vi "PrefDialog.vi"(8 "error in (no error)":errorcluster, 11 "MyPluginsBase in":refnum<class "PacificPowerSource.lvclass">) -> (0 "error out":errorcluster, 1 "Save As":bool, 2 "Changed":bool, 3 "MyPluginsBase out":refnum<class "PacificPowerSource.lvclass">)   [LabVIEW 2018, in "AcPwrPlugins.lvlib" / "PacificPowerSource.lvclass"]
doc: "This VI allows the user to display the previous instrument's settings, change these settings, and save the current settings to the same file or a new file with a new \"Type\" identifier."
uses:
  PacificPowerSource.lvclass
  C:/Program Files (x86)/National Instruments/LabVIEW 2018/user.lib/NIST/BaseClasses/BasePlugin_class/BasePlugin.lvclass
  C:/Users/ico/Documents/Projects/NistPluggableModules/AcPwr/AcPwrPlugins/AcPwrBaseClass/AcPwrBase.lvclass
  TypeDefs/Device(s)Settings.ctl
  AcPwrBaseClass/TypeDefs/BaseMeasurements.ctl
  ChromaAcLoadClass/TypeDefs/MeasurementType.ctl
  TypeDefs/Measurements.ctl
  TypeDefs/MeasurementType.ctl
  <userlib>/NIST/BaseClasses/BasePlugin_class/BasePlugin.lvclass/BasePlugin.ctl
  AcPwrBaseClass/AcPwrBase.lvclass/AcPwrBase.ctl
  <userlib>/NIST/BaseClasses/BasePlugin_class/Accessors/Read PluginIniFilePath.vi
  AcPwrBaseClass/Accessors/Read BaseConfig.vi
  AcPwrBaseClass/Accessors/Read BaseMeasurements.vi
  <userlib>/NIST/BaseClasses/BasePlugin_class/Accessors/Write PluginIniFilePath.vi
  <vilib>/Utility/config.llb/NI_LVConfig.lvlib
  AcPwrBaseClass/AcPwrBase.lvclass
  ChromaAcLoadClass/ChromaAcLoad.lvclass
panel:
  in  "Measurements":T1
  in  "BaseMeasurements":T3 {"NHRGridSim Phase" items=["All", "A Phase", "B Phase", "C Phase"]; "NHRDC Measurement Type" items=["Voltage"=1, "Positive Peak Voltage"=2, "Positive Peak Voltage Last Fetch"=4, "Negative Peak Voltage"=8, "Negative Peak Voltage Last Fetch"=16, "Current"=32, "Positive Peak Current"=64, "Positive Peak Current Last Fetch"=128, "Negative Peak Current"=256, "Negative Peak Current Last Fetch"=512, "Power"=1024, "Positive Peak Power"=2048, "Positive Peak Power Last Fetch"=4096, "Negative Peak Power"=8192, "Negative Peak Power Last Fetch"=16384, "Timestamp"=32768, "Charge Time"=65536, "Discharge Time"=131072, "Amp Hour"=262144, "Amp Hour Time"=524288, "Amp Hour Charge"=1048576, "Amp Hour Discharge"=2097152, "Kilo Watt Hour"=4194304, "Kilo Watt Hour Time"=8388608, "Kilo Watt Hour Charge"=16777216, "Kilo Watt Hour Discharge"=33554432, "UUT Temperature"=67108864]; "NHRDC Fetch Method" items=["Aperture", "Immediate"]}
  in  "btnSaveAs":bool
  in  "Measurement RefreshTime (ms)":u32
  in  "btnSave":bool
  in  "btnCancel":bool
  in  "Device(s)Settings":T5 {"Modules"."Source Range"."Frequency Range (600Hz)" items=["150 Hz", "300 Hz", "600 Hz", "1200 Hz"]; "Modules"."Source Range"."Range Control (0: Auto)" items=["Auto", "<110 V", "110 V -120.9 V", "121 V - 130.9 V", "> 131 V"]; "Modules"."Program #"."Waveform C (1: Sine)" items=["Sine"=1, "Arbitrary Waveform 2"=2, "Arbitrary Waveform 3"=3, "Arbitrary Waveform 4"=4, "Arbitrary Waveform 5"=5, "Arbitrary Waveform 6"=6, "Arbitrary Waveform 7"=7, "Arbitrary Waveform 8"=8, "Arbitrary Waveform 9"=9, "Arbitrary Waveform 10"=10, "Arbitrary Waveform 11"=11, "Arbitrary Waveform 12"=12, "Arbitrary Waveform 13"=13, "Arbitrary Waveform 14"=14, "Arbitrary Waveform 15"=15, "Arbitrary Waveform 16"=16, "Arbitrary Waveform 17"=17, "Arbitrary Waveform 18"=18, "Arbitrary Waveform 19"=19, "Arbitrary Waveform 20"=20, "Arbitrary Waveform 21"=21, "Arbitrary Waveform 22"=22]; "Modules"."Program #"."Waveform B (1: Sine)" items=["Sine"=1, "Arbitrary Waveform 2"=2, "Arbitrary Waveform 3"=3, "Arbitrary Waveform 4"=4, "Arbitrary Waveform 5"=5, "Arbitrary Waveform 6"=6, "Arbitrary Waveform 7"=7, "Arbitrary Waveform 8"=8, "Arbitrary Waveform 9"=9, "Arbitrary Waveform 10"=10, "Arbitrary Waveform 11"=11, "Arbitrary Waveform 12"=12, "Arbitrary Waveform 13"=13, "Arbitrary Waveform 14"=14, "Arbitrary Waveform 15"=15, "Arbitrary Waveform 16"=16, "Arbitrary Waveform 17"=17, "Arbitrary Waveform 18"=18, "Arbitrary Waveform 19"=19, "Arbitrary Waveform 20"=20, "Arbitrary Waveform 21"=21, "Arbitrary Waveform 22"=22]; "Modules"."Program #"."Coupling  (0: Direct)" items=["Direct", "Transformer"]; "Modules"."Program #"."Form (3: Three)" items=["Single", "Split", "Three"]; "Modules"."Program #"."Program Number (0)" min=1; "Modules"."Program #"."Waveform A (1: Sine)" items=["Sine"=1, "Arbitrary Waveform 2"=2, "Arbitrary Waveform 3"=3, "Arbitrary Waveform 4"=4, "Arbitrary Waveform 5"=5, "Arbitrary Waveform 6"=6, "Arbitrary Waveform 7"=7, "Arbitrary Waveform 8"=8, "Arbitrary Waveform 9"=9, "Arbitrary Waveform 10"=10, "Arbitrary Waveform 11"=11, "Arbitrary Waveform 12"=12, "Arbitrary Waveform 13"=13, "Arbitrary Waveform 14"=14, "Arbitrary Waveform 15"=15, "Arbitrary Waveform 16"=16, "Arbitrary Waveform 17"=17, "Arbitrary Waveform 18"=18, "Arbitrary Waveform 19"=19, "Arbitrary Waveform 20"=20, "Arbitrary Waveform 21"=21, "Arbitrary Waveform 22"=22]}
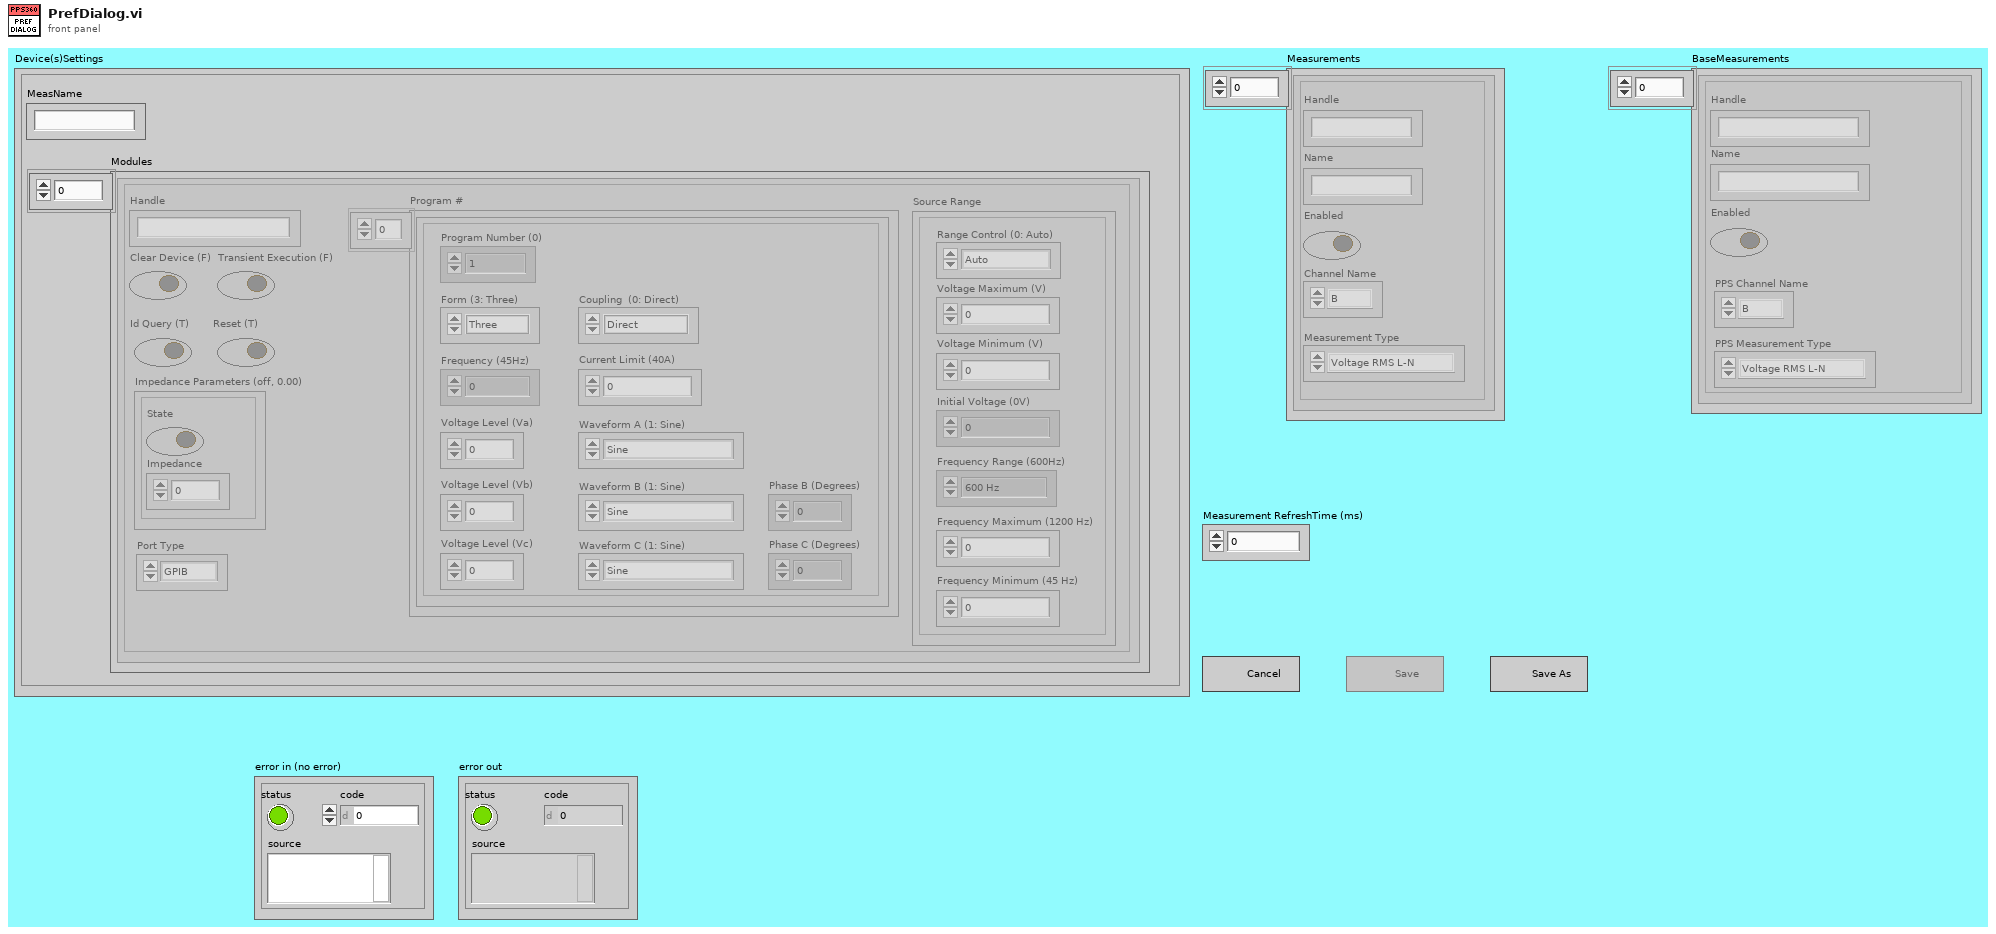
[diagram p1: front panel]
types:
  T1 = typedef "AcPwrPlugins.lvlib/PacificPowerSource.lvclass/Measurements.ctl" = cluster{"Handle":string, "Name":string, "Enabled ":bool, "Measurement Value":dbl, "Channel Name":enum16{"A", "B", "C"}, "Measurement Type ":T2}[]
  T2 = typedef "AcPwrPlugins.lvlib/PacificPowerSource.lvclass/MeasurementType.ctl" = enum16{"Voltage RMS L-N", "Voltage RMS L-L", "Frequency", "Current RMS", "Current Peak", "Crest Factor", "Power Factor", "Power VA", "Real Power"}
  T3 = typedef "AcPwrPlugins.lvlib/AcPwrBase.lvclass/BaseMeasurements.ctl" = cluster{"Handle":string, "Name":string, "Enabled":bool, "Measurement Value":dbl, "btnMeasFetch":bool, "Chroma Hold Peak Current Measurement":bool, "Chroma Measurement Type":T4, "Chroma Protection Status String":string, "NHRDC Fetch Method":i32, "NHRDC Fetch Time (s)":sgl, "NHRDC Measurement Type":i32, "NHRGridSim Measurement Type ":enum16{"Average Current", "Max Current", "Min Current", "Average Voltage", "Max Voltage", "Min Voltage", "Average True Power", "Max True Power", "Min True Power", "Average Apparent Power", "Max Apparent Power", "Min Apparent Power", "Power Factor", "Crest Factor"}, "NHRGridSim Phase ":i32, "PPS Measurement Type ":enum16{"Voltage RMS L-N", "Voltage RMS L-L", "Frequency", "Current RMS", "Current Peak", "Crest Factor", "Power Factor", "Power VA", "Real Power"}, "PPS Channel Name":enum16{"A", "B", "C"}}[]
  T4 = typedef "AcPwrPlugins.lvlib/ChromaAcLoad.lvclass/MeasurementType.ctl" = enum16{"Voltage (Vrms or V)", "Current (Arms or A)", "Power (W)", "Peak Voltage (V)", "Peak Current (A)", "Peak Power (W)", "Frequency (Hz)", "Resistance (Ohms)", "Voltage Overshoot (V)", "Positive Peak Current (A)", "Voltage Undershoot (V)", "Negative Peak Current (A)", "Apparent Power (VA)", "Reacitive Power (VAR)", "Voltage THD", "Power Factor", "Current's Crest Factor"}
  T5 = typedef "AcPwrPlugins.lvlib/PacificPowerSource.lvclass/Device(s)Settings.ctl" = cluster{"MeasName":string, "Modules":cluster{"Handle":string, "Connected":bool, "Clear Device (F)":bool, "btnIdQuery":bool, "btnReset":bool, "Program #":cluster{"Phase B (Degrees)":i32, "Waveform A (1: Sine)":i32, "Voltage Level (Va)":dbl, "Program Number (0)":i32, "Voltage Level (Vb) ":dbl, "Form (3: Three)":u16, "Coupling  (0: Direct)":u16, "Frequency (45Hz)":dbl, "Current Limit (40A)":dbl, "Phase C (Degrees)":i32, "Voltage Level (Vc)":dbl, "Waveform B (1: Sine)":i32, "Waveform C (1: Sine)":i32}[], "Impedance Parameters (off, 0.00)":cluster{"State":bool, "Impedance":dbl}, "Transient Execution (F)":bool, "OutputEnabled":bool, "Source Range":cluster{"Frequency Minimum (45 Hz)":dbl, "Frequency Maximum (1200 Hz)":dbl, "Voltage Maximum (V)":dbl, "Voltage Minimum (V)":dbl, "Range Control (0: Auto)":u16, "Initial Voltage (0V)":u16, "Frequency Range (600Hz)":u16}, "Port Type":enum16{"GPIB", "Serial"}}[]}
  T6 = enum32{"Invalid", "Standard", "Closed", "Hidden", "Minimized", "Maximized"}
  T7 = enum32{"Invalid", "Default", "Floating", "Floating/Auto-Hide", "Modal"}
  T8 = enum8{"Enabled", "Disabled", "Disabled and Grayed Out"}
  T9 = typedef "AcPwrPlugins.lvlib/PacificPowerSource.lvclass/Modules.ctl" = cluster{"Handle":string, "Connected":bool, "Clear Device (F)":bool, "btnIdQuery":bool, "btnReset":bool, "Program #":cluster{"Phase B (Degrees)":i32, "Waveform A (1: Sine)":i32, "Voltage Level (Va)":dbl, "Program Number (0)":i32, "Voltage Level (Vb) ":dbl, "Form (3: Three)":u16, "Coupling  (0: Direct)":u16, "Frequency (45Hz)":dbl, "Current Limit (40A)":dbl, "Phase C (Degrees)":i32, "Voltage Level (Vc)":dbl, "Waveform B (1: Sine)":i32, "Waveform C (1: Sine)":i32}[], "Impedance Parameters (off, 0.00)":cluster{"State":bool, "Impedance":dbl}, "Transient Execution (F)":bool, "OutputEnabled":bool, "Source Range":cluster{"Frequency Minimum (45 Hz)":dbl, "Frequency Maximum (1200 Hz)":dbl, "Voltage Maximum (V)":dbl, "Voltage Minimum (V)":dbl, "Range Control (0: Auto)":u16, "Initial Voltage (0V)":u16, "Frequency Range (600Hz)":u16}, "Port Type":enum16{"GPIB", "Serial"}}[]
  T10 = cluster{"Handle":string, "Connected":bool, "Clear Device (F)":bool, "btnIdQuery":bool, "btnReset":bool, "Program #":cluster{"Phase B (Degrees)":i32, "Waveform A (1: Sine)":i32, "Voltage Level (Va)":dbl, "Program Number (0)":i32, "Voltage Level (Vb) ":dbl, "Form (3: Three)":u16, "Coupling  (0: Direct)":u16, "Frequency (45Hz)":dbl, "Current Limit (40A)":dbl, "Phase C (Degrees)":i32, "Voltage Level (Vc)":dbl, "Waveform B (1: Sine)":i32, "Waveform C (1: Sine)":i32}[], "Impedance Parameters (off, 0.00)":cluster{"State":bool, "Impedance":dbl}, "Transient Execution (F)":bool, "OutputEnabled":bool, "Source Range":cluster{"Frequency Minimum (45 Hz)":dbl, "Frequency Maximum (1200 Hz)":dbl, "Voltage Maximum (V)":dbl, "Voltage Minimum (V)":dbl, "Range Control (0: Auto)":u16, "Initial Voltage (0V)":u16, "Frequency Range (600Hz)":u16}, "Port Type":enum16{"GPIB", "Serial"}}[]
  T11 = cluster{"Handle":string, "Connected":bool, "Clear Device (F)":bool, "btnIdQuery":bool, "btnReset":bool, "Program #":cluster{"Phase B (Degrees)":i32, "Waveform A (1: Sine)":i32, "Voltage Level (Va)":dbl, "Program Number (0)":i32, "Voltage Level (Vb) ":dbl, "Form (3: Three)":u16, "Coupling  (0: Direct)":u16, "Frequency (45Hz)":dbl, "Current Limit (40A)":dbl, "Phase C (Degrees)":i32, "Voltage Level (Vc)":dbl, "Waveform B (1: Sine)":i32, "Waveform C (1: Sine)":i32}[], "Impedance Parameters (off, 0.00)":cluster{"State":bool, "Impedance":dbl}, "Transient Execution (F)":bool, "OutputEnabled":bool, "Source Range":cluster{"Frequency Minimum (45 Hz)":dbl, "Frequency Maximum (1200 Hz)":dbl, "Voltage Maximum (V)":dbl, "Voltage Minimum (V)":dbl, "Range Control (0: Auto)":u16, "Initial Voltage (0V)":u16, "Frequency Range (600Hz)":u16}, "Port Type":enum16{"GPIB", "Serial"}}
  T12 = typedef "AcPwrPlugins.lvlib/AcPwrBase.lvclass/BaseConfig.ctl" = cluster{"Frequency":dbl, "FrequencyRange":dbl[], "Phases":T13[], "Name":string, "PluginConfigVariant":variant, "PluginMeasVariant":variant}
  T13 = typedef "AcPwrPlugins.lvlib/AcPwrBase.lvclass/Phase.ctl" = cluster{"Name":string, "Enabled":bool, "VoltageLevel":dbl, "Handle":string, "VoltageRange":dbl[], "Connected":bool, "CurrentLimit":dbl, "Waveform":string}
  T14 = typedef "NI_LVConfig.lvlib/Config Data RefNum.ctl" = refnum<k1>
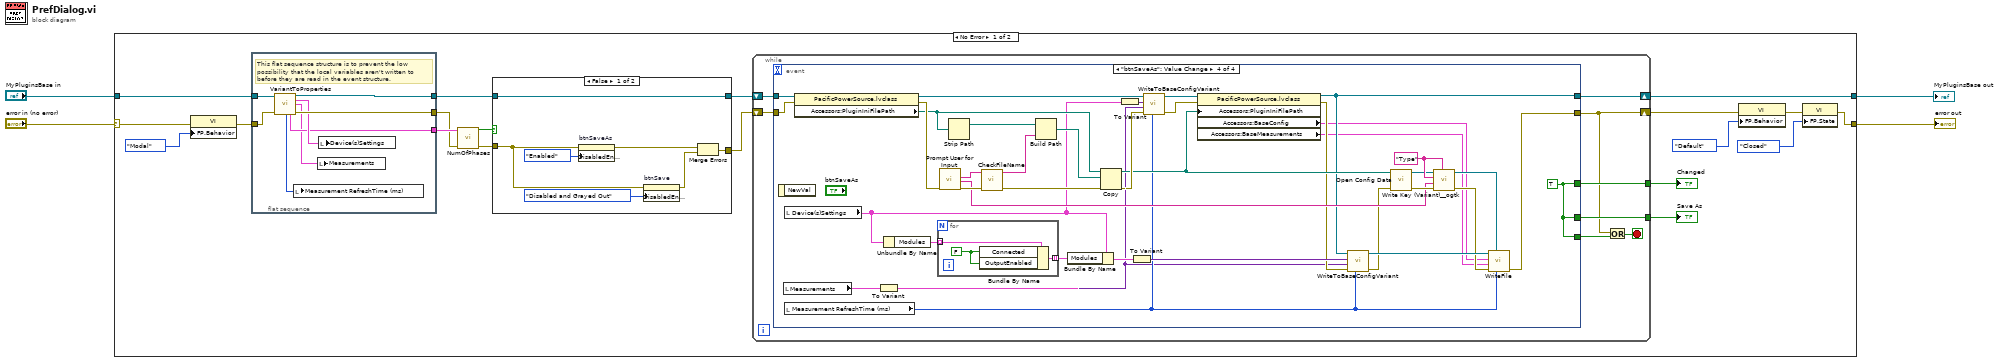
[diagram p0: block diagram]
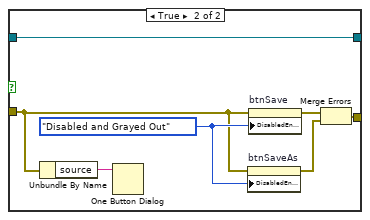
[diagram p2: hidden frame]
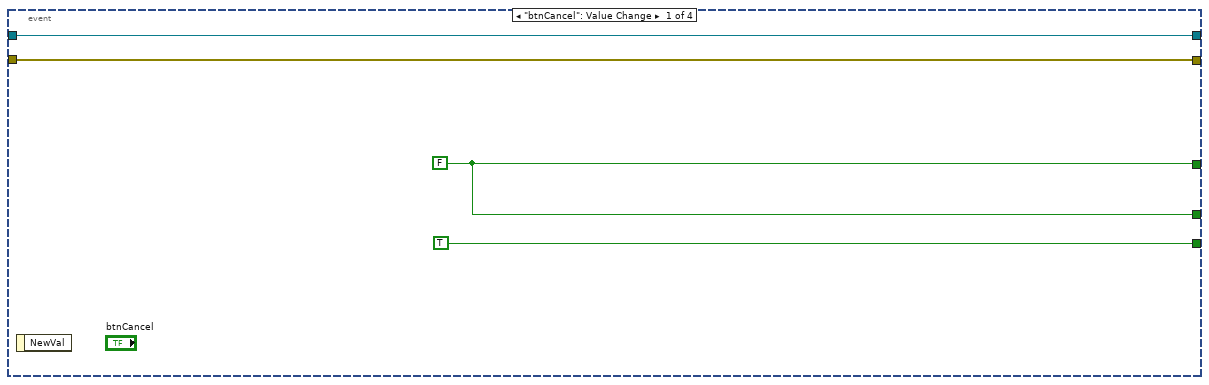
[diagram p3: hidden frame]
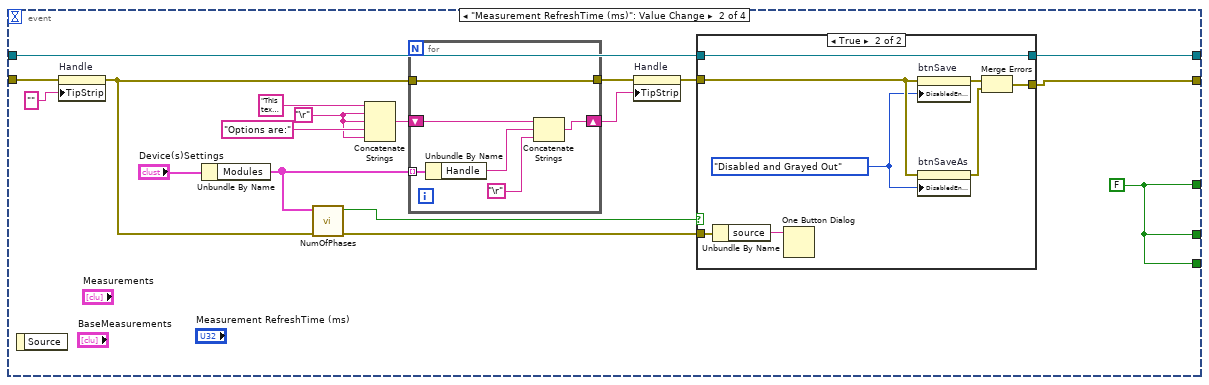
[diagram p4: hidden frame]
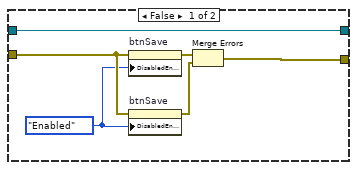
[diagram p5: hidden frame]
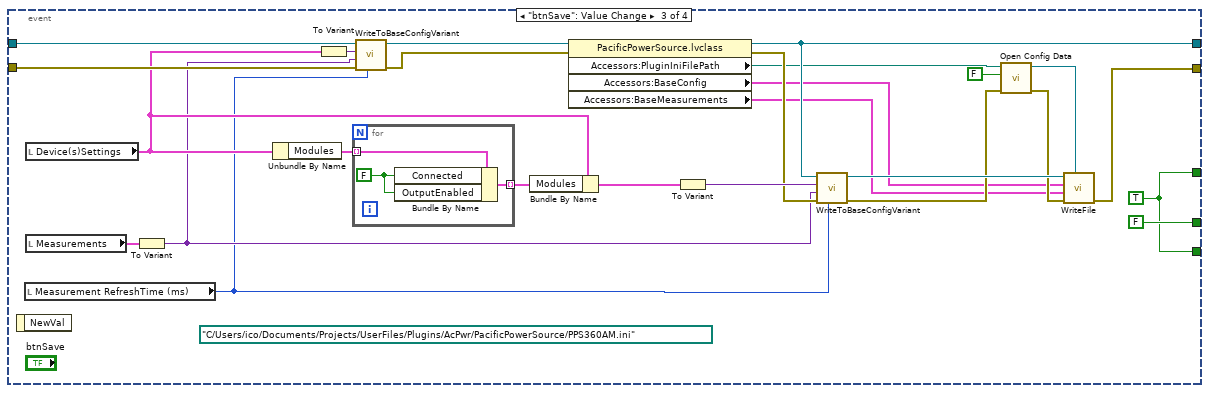
[diagram p6: hidden frame]
diagram:
  n1 = case shown="No Error" "error in (no error)" {
    selector: "error in (no error)" -> [w22 w167]
    tunnel: "MyPluginsBase in" -> [w17 w166]
    tunnel: [w16 w166] -> w2
    tunnel: [w15 w167] -> w1
    frame No Error {
      n2 = property class="VI"(error in=w22, "FP.Behavior"=T7."Modal" ("Front Panel Window:Behavior")) -> (error out=w18:errorcluster)  [unwired: 1 in, 1 out]
      n3 = flat-sequence {
        tunnel: w17 -> [w31]
        tunnel: [w29] -> w6
        tunnel: [w28] -> w7
        tunnel: w18 -> [w30]
        tunnel: [w25] -> w10
        frame #0 {
          # "This flat sequence structure is to prevent the low possibility that the local variables aren't written to before they are read in the event structure."
          n4 = call "VariantToProperties.vi"("PacificPowerSource in"=w31, "error in (no error)"=w30) -> ("PacificPowerSource out"=w29:refnum<class "PacificPowerSource.lvclass">, "Device(s)Settings"=w27:T5, "Measurements"=w24:T1, "Measurement Refresh Time (ms)"=w26:u32, "Modules"=w25:T9, "error out"=w28:errorcluster)  [unwired: 7 in, 1 out]
          n5 = local write "Measurement RefreshTime (ms)"(w26) -> ()
          n6 = local write "Measurements"(w24) -> ()
          n7 = local write "Device(s)Settings"(w27) -> ()
        }
      }
      n8 = call "NumOfPhases.vi"("Error In"=w7, "Modules"=w10) -> ("Error Out"=w8:errorcluster, "NumberOfPhases>3"=w9:bool)  [unwired: 7 in, 1 out]
      n9 = case shown="False" w9 {
        tunnel: [w37 w44] -> w11
        tunnel: w8 -> [w33 w40]
        tunnel: w6 -> [w32 w39]
        tunnel: [w32 w39] -> w5
        frame False {
          # "Check if the number of Phases=Loads. If no disables the ability\nto save as."
          n10 = property on="btnSaveAs" class="Bool"(error in=w33, "DisabledEnum"=T8."Enabled" ("Disabled")) -> (error out=w38:errorcluster)  [unwired: 1 in, 1 out]
          n11 = property on="btnSave" class="Bool"(error in=w33, "DisabledEnum"=T8."Disabled and Grayed Out" ("Disabled")) -> (error out=w36:errorcluster)  [unwired: 1 in, 1 out]
          n12 = Merge Errors(w38, w36) -> (w37:errorcluster)
        }
        frame True {
          w42 = T8."Disabled and Grayed Out" ("Disabled")
          # "Check if the number of Phases=Loads. If no disables the ability\nto save as."
          n13 = Unbundle By Name(w40) -> ("source"=w41:string)
          n14 = One Button Dialog(message=w41) -> ()  [unwired: 1 in, 1 out]
          n15 = property on="btnSaveAs" class="Bool"(error in=w40, "DisabledEnum"=w42) -> (error out=w43:errorcluster)  [unwired: 1 in, 1 out]
          n16 = property on="btnSave" class="Bool"(error in=w40, "DisabledEnum"=w42) -> (error out=w45:errorcluster)  [unwired: 1 in, 1 out]
          n17 = Merge Errors(w45, w43) -> (w44:errorcluster)
        }
      }
      n18 = while {
        shift-right: [w50] -> w16
        shift-left: w5 -> [w51]
        tunnel: [w53] -> w13
        tunnel: [w48] -> w12
        shift-right: [w46] -> w14
        shift-left: w11 -> [w49]
        stop <- w47 stop-if-true
        n19 = event shown="[3] \"btnSaveAs\": Value Change" {
          selector: _ -> [_ _ _ _]
          dyn-events: _ -> [_ _ _ _]
          timeout: _ -> [_ _ _ _]
          tunnel: [w54 w75 w120 w160] -> w53
          tunnel: [TRUE w75 w120 w160] -> w52
          tunnel: w51 -> [w56 w62 w115 w152]
          tunnel: [w56 w63 w105 w132] -> w50
          tunnel: [w55 w74 w119 w146] -> w46
          tunnel: w49 -> [w55 w72 w114 w151]
          tunnel: [w54 w75 FALSE w160] -> w48
          event "btnCancel": Value Change {
            w54 = FALSE
            n20 = event-data() -> ()  [unwired: 1 in, 1 out]
          }
          event "Measurement RefreshTime (ms)": Value Change {
            w68 = "\r"
            w75 = FALSE
            n21 = event-data() -> ()  [unwired: 1 in, 1 out]
            n22 = property on="Handle" class="Str"(error in=w72, "TipStrip"="" ("Tip Strip")) -> (error out=w61:errorcluster)  [unwired: 1 in, 1 out]
            n23 = Unbundle By Name("Device(s)Settings") -> ("Modules"=w58:T10)
            n24 = call "NumOfPhases.vi"("Error In"=w61, "Modules"=w58) -> ("Error Out"=w65:errorcluster, "NumberOfPhases>3"=w59:bool)  [unwired: 7 in, 1 out]
            n25 = Concatenate Strings("This text in this handle of the instrument and entered in the  \nhandle control in the Phases array EXACTLY, lest the attempt \nto interact with the instrument will fail.", w68, w68, "Options are:" ("Handle"), w68) -> (w67:string)
            n26 = for {
              shift-right: [w81] -> w66
              shift-left: w67 -> [w80]
              tunnel: w58 -> [w79] mode=indexing
              tunnel: w61 -> [w76]
              tunnel: [w76] -> w60
              n27 = Unbundle By Name(w79) -> ("Handle"=w78:string)
              n28 = Concatenate Strings(w80, w78, "\r") -> (w81:string)
            }
            n29 = property on="Handle" class="Str"(error in=w60, "TipStrip"=w66) -> (error out=w73:errorcluster)  [unwired: 1 in, 1 out]
            n30 = case shown="True" w59 {
              tunnel: w73 -> [w86 w94]
              tunnel: [w85 w93] -> w74
              tunnel: w65 -> [_ w89]
              tunnel: w62 -> [w82 w88]
              tunnel: [w82 w88] -> w63
              frame False {
                w83 = T8."Enabled" ("Disabled")
                # "Check if the number of Phases=Loads. If no disables the ability\nto save as."
                n31 = property on="btnSave" class="Bool"(error in=w86, "DisabledEnum"=w83) -> (error out=w87:errorcluster)  [unwired: 1 in, 1 out]
                n32 = property on="btnSave" class="Bool"(error in=w86, "DisabledEnum"=w83) -> (error out=w84:errorcluster)  [unwired: 1 in, 1 out]
                n33 = Merge Errors(w87, w84) -> (w85:errorcluster)
              }
              frame True {
                w91 = T8."Disabled and Grayed Out" ("Disabled")
                # "Check if the number of Phases=Loads. If no disables the ability\nto save as."
                n34 = Unbundle By Name(w89) -> ("source"=w90:string)
                n35 = One Button Dialog(message=w90) -> ()  [unwired: 1 in, 1 out]
                n36 = property on="btnSave" class="Bool"(error in=w94, "DisabledEnum"=w91) -> (error out=w95:errorcluster)  [unwired: 1 in, 1 out]
                n37 = property on="btnSaveAs" class="Bool"(error in=w94, "DisabledEnum"=w91) -> (error out=w92:errorcluster)  [unwired: 1 in, 1 out]
                n38 = Merge Errors(w95, w92) -> (w93:errorcluster)
              }
            }
          }
          event "btnSave": Value Change {
            (unwired) path "C:/Users/ico/Documents/Projects/UserFiles/Plugins/AcPwr/PacificPowerSource/PPS360AM.ini" ("configuration file path")
            w120 = TRUE ("StartMeas")
            n39 = event-data() -> ()  [unwired: 1 in, 1 out]
            n40 = local read "Measurement RefreshTime (ms)"() -> (w97:u32)
            n41 = local read "Device(s)Settings"() -> (w113:T5)
            n42 = local read "Measurements"() -> (w99:T1)
            n43 = To Variant(anything=w99) -> (Variant=w98:variant)
            n44 = Unbundle By Name(w113) -> ("Modules"=w112:T10)
            n45 = To Variant(anything=w113) -> (Variant=w118:variant)
            n46 = for {
              tunnel: w112 -> [w124] mode=indexing
              tunnel: [w123] -> w109 mode=indexing
              w122 = FALSE ("Connected")
              n47 = Bundle By Name(cluster=w124, "Connected"=w122, "OutputEnabled"=w122) -> (w123:T11)
            }
            n48 = call "WriteToBaseConfigVariant.vi"("Measurement Refresh Time (ms)"=w97, "error in (no error)"=w114, "Meas"=w98, "Config"=w118, "PacificPowerSource in"=w115) -> ("error out"=w116:errorcluster, "PacificPowerSource out"=w117:refnum<class "PacificPowerSource.lvclass">)  [unwired: 5 in]
            n49 = Bundle By Name(cluster=w113, "Modules"=w109) -> (w102:T5)
            n50 = property class="PacificPowerSource.lvclass"(reference=w117, error in=w116) -> (reference out=w105:refnum<class "PacificPowerSource.lvclass">, error out=w108:errorcluster, "Accessors:PluginIniFilePath"=w101:path, "Accessors:BaseConfig"=w100:T12, "Accessors:BaseMeasurements"=w96:T3)
            n51 = To Variant(anything=w102) -> (Variant=w110:variant)
            n52 = call "WriteToBaseConfigVariant.vi"("Measurement Refresh Time (ms)"=w97, "error in (no error)"=w108, "Meas"=w98, "Config"=w110, "PacificPowerSource in"=w105) -> ("error out"=w106:errorcluster, "PacificPowerSource out"=w107:refnum<class "PacificPowerSource.lvclass">)  [unwired: 5 in]
            n53 = call <vilib>:"Open Config Data.vi"("error in (no error)"=w106, "create file if necessary (T)"=FALSE, "configuration file path"=w101) -> ("error out"=w104:errorcluster, "refnum"=w103:T14)  [unwired: 6 in, 1 out]
            n54 = call-dynamic "WriteFile.vi"("Refnum in"=w103, "error in (no error)"=w104, "BaseMeasurements"=w96, "BaseConfiguration"=w100, "PacificPowerSource in"=w107) -> ("error out"=w119:errorcluster)  [unwired: 5 in, 1 out]
          }
          event "btnSaveAs": Value Change {
            w156 = "Type" ("section (optional)")
            w160 = TRUE
            n55 = event-data() -> ()  [unwired: 1 in, 1 out]
            n56 = local read "Measurements"() -> (w126:T1)
            n57 = local read "Device(s)Settings"() -> (w136:T5)
            n58 = local read "Measurement RefreshTime (ms)"() -> (w128:u32)
            n59 = property class="PacificPowerSource.lvclass"(reference=w152, error in=w151) -> (reference out=w142:refnum<class "PacificPowerSource.lvclass">, error out=w150:errorcluster, "Accessors:PluginIniFilePath"=w148:path)
            n60 = To Variant(anything=w126) -> (Variant=w125:variant)
            n61 = Unbundle By Name(w136) -> ("Modules"=w144:T10)
            n62 = for {
              tunnel: w144 -> [w165] mode=indexing
              tunnel: [w164] -> w147 mode=indexing
              w163 = FALSE ("Connected")
              n63 = Bundle By Name(cluster=w165, "Connected"=w163, "OutputEnabled"=w163) -> (w164:T11)
            }
            n64 = call "Prompt User for Input"("error in (no error)"=w150) -> ("File Name"=w149:string, "PluginType"=w153:string, "error out"=w157:errorcluster)  [unwired: 15 in, 1 out]
            n65 = Strip Path(path=w148) -> (stripped path=w162:path)  [unwired: 1 out]
            n66 = call "CheckFileName.vi"("Error In"=w157, "File Name in"=w149) -> ("Error Out"=w158:errorcluster, "File Name out"=w159:string)  [unwired: 8 in]
            n67 = Build Path(base path=w162, name or relative path=w159) -> (appended path=w161:path)
            n68 = Bundle By Name(cluster=w136, "Modules"=w147) -> (w135:T5)
            n69 = Copy(8:w158, 10:w161, 11:w148) -> (0:w139:errorcluster, 3:w138:path)  [unwired: 2 in, 1 out]
            n70 = To Variant(anything=w136) -> (Variant=w143:variant)
            n71 = To Variant(anything=w135) -> (Variant=w137:variant)
            n72 = call "WriteToBaseConfigVariant.vi"("Measurement Refresh Time (ms)"=w128, "error in (no error)"=w139, "Meas"=w125, "Config"=w143, "PacificPowerSource in"=w142) -> ("error out"=w140:errorcluster, "PacificPowerSource out"=w141:refnum<class "PacificPowerSource.lvclass">)  [unwired: 5 in]
            n73 = property class="PacificPowerSource.lvclass"(reference=w141, error in=w140, "Accessors:PluginIniFilePath"=w138) -> (reference out=w132:refnum<class "PacificPowerSource.lvclass">, error out=w133:errorcluster, "Accessors:BaseConfig"=w129:T12, "Accessors:BaseMeasurements"=w127:T3)
            n74 = call "WriteToBaseConfigVariant.vi"("Measurement Refresh Time (ms)"=w128, "error in (no error)"=w133, "Meas"=w125, "Config"=w137, "PacificPowerSource in"=w132) -> ("error out"=w131:errorcluster, "PacificPowerSource out"=w134:refnum<class "PacificPowerSource.lvclass">)  [unwired: 5 in]
            n75 = call <vilib>:"Open Config Data.vi"("error in (no error)"=w131, "configuration file path"=w138) -> ("error out"=w154:errorcluster, "refnum"=w155:T14)  [unwired: 7 in, 1 out]
            n76 = call <userlib>:"Write Key (Variant)__ogtk.vi"("section"=w156, "error in (no error)"=w154, "key-value"=w153, "key (optional)"=w156, "refnum"=w155) -> ("error out"=w130:errorcluster, "refnum out"=w145:T14)  [unwired: 5 in]
            n77 = call-dynamic "WriteFile.vi"("RefreshTime"=w128, "Refnum in"=w145, "error in (no error)"=w130, "BaseMeasurements"=w127, "BaseConfiguration"=w129, "PacificPowerSource in"=w134) -> ("error out"=w146:errorcluster)  [unwired: 4 in, 1 out]
          }
        }
        n78 = Or(x=w46, y=w52) -> (x .or. y?=w47:bool)
      }
      "Save As" <- w12
      "Changed" <- w13
      n79 = property class="VI"(error in=w14, "FP.Behavior"=T7."Default" ("Front Panel Window:Behavior")) -> (error out=w21:errorcluster)  [unwired: 1 in, 1 out]
      n80 = property class="VI"(error in=w21, "FP.State"=T6."Closed" ("Front Panel Window:State")) -> (error out=w15:errorcluster)  [unwired: 1 in, 1 out]
    }
    frame Error {
    }
  }
  "error out" <- w1
  "MyPluginsBase out" <- w2
